vi "UDPsender Rigid Joystick.vi"(11 "nums2send":dbl[](array[numeric])=[0.0, 0.0, 0.0, 0.0]) -> (3 "string2send":string)   [LabVIEW 2016]
panel:
  # "x actual [mm]"
  # "y actual [mm]"
  # ">>>"
  # "z actual [mm]"
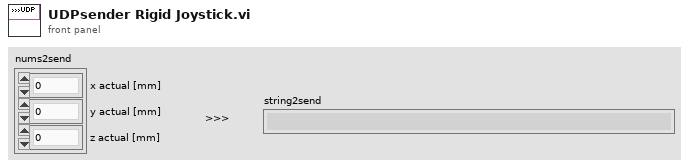
[diagram p1: front panel]
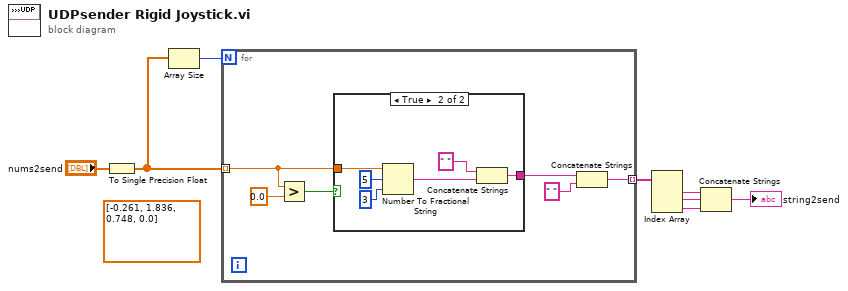
[diagram p0: block diagram]
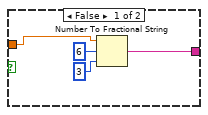
[diagram p2: hidden frame]
diagram:
  (unwired) dbl[] [-0.261, 1.836, 0.748, 0.0] ("nums2send 2")
  n1 = To Single Precision Float(number="nums2send") -> (single precision float=w1:sgl[])
  n2 = Array Size(array=w1) -> (size(s)=w7:i32)
  n3 = for {
    N: w7 -> [_]
    tunnel: w1 -> [w12] mode=indexing
    tunnel: [w11] -> w6 mode=indexing
    n4 = Greater?(x=w12, y=0.0) -> (0:w13:bool)
    n5 = case shown="True" w13 {
      tunnel: [w15 w19] -> w9
      tunnel: w12 -> [w16 w20]
      frame False {
        n6 = Number To Fractional String(number=w16, width (-)=i16 6, precision (6)=i16 3) -> (F-format string=w15:string)  [unwired: 1 out]
      }
      frame True {
        n7 = Number To Fractional String(number=w20, width (-)=i16 5, precision (6)=i16 3) -> (F-format string=w22:string)  [unwired: 1 out]
        n8 = Concatenate Strings(" " ("string"), w22) -> (w19:string)
      }
    }
    n9 = Concatenate Strings(w9, " " ("string")) -> (w11:string)
  }
  n10 = Index Array(array=w6) -> (element #1=w5:string, element #2=w4:string, element #3=w3:string)  [unwired: 3 in]
  n11 = Concatenate Strings(w5, w4, w3) -> (→"string2send":string)
